vi "Handle.vi"(11 "jettl Event Actor in":refnum<class "jettl Event Actor.lvclass">) -> (2 "Destroy?":bool, 3 "jettl Event Actor out":refnum<class "jettl Event Actor.lvclass">)   [LabVIEW 2021, in "jettl.lvlib" / "jettl Event Actor.lvclass"]
uses:
  jettl Event Actor.lvclass
  C:/git/jettl/src/Actor/Event Actor/Event Actor.lvclass
  jettl Event Actor.lvclass/jettl Event Actor.ctl
  Event State/Event State/Event State.lvclass
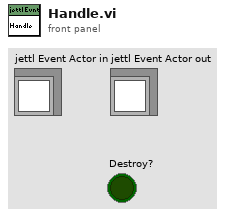
[diagram p1: front panel]
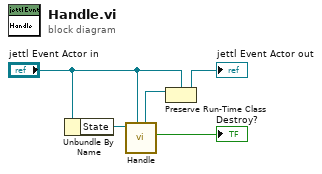
[diagram p0: block diagram]
diagram:
  n1 = Unbundle By Name("jettl Event Actor in") -> ("State"=w4:refnum<class "Event State.lvclass">)
  n2 = call-dynamic "Handle.vi"("Event Actor in"="jettl Event Actor in", "Event State in"=w4) -> ("Destroy?"=→"Destroy?":bool, "Event Actor out"=w2:refnum<class "Event Actor.lvclass">)  [unwired: 8 in]
  n3 = Preserve Run-Time Class(object in=w2, 2:"jettl Event Actor in") -> (object out=→"jettl Event Actor out":refnum<class "jettl Event Actor.lvclass">)  [unwired: 1 in, 1 out]
